vi "Offset Two Points Rectangle by Array Pointer.vi"() -> ()   [LabVIEW 2012]
uses:
  demo dll.dll
panel:
  out "OffsetRect":i32[](array[numeric])=[4, 10, 14, 40]
  in  "TwoPointsRect":i32[](array[numeric])=[0, 0, 10, 30]
  in  "Point":cluster{"x":i32, "y":i32}={"x"=4, "y"=10}
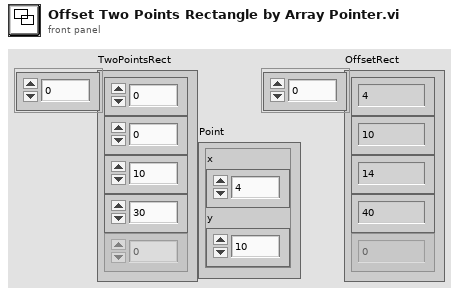
[diagram p1: front panel]
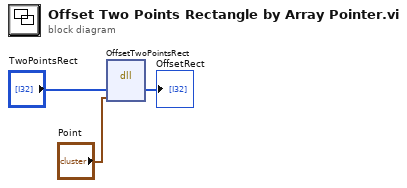
[diagram p0: block diagram]
diagram:
  n1 = dll-call lib="PTH1+abs EBOOK\t功能块DLLdemo dll.dll" fn="OffsetTwoPointsRect"("Rect"="TwoPointsRect", "OffPoint"="Point") -> ("Rect"=→"OffsetRect":i32[])  [unwired: 5 in, 2 out]
